vi "GEA3 HexStringToBoolean.vi"(2 "Hex String":string) -> (0 "Boolean":bool, 1 "decimal integer string":string)   [LabVIEW 2020]
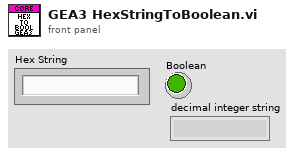
[diagram p1: front panel]
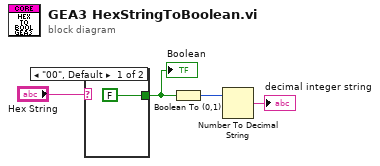
[diagram p0: block diagram]
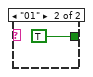
[diagram p2: hidden frame]
diagram:
  n1 = case shown="\"00\", Default" "Hex String" {
    tunnel: [FALSE ("Eco Wash") TRUE ("Eco Wash")] -> w3
    frame "00", Default {
    }
    frame "01" {
    }
  }
  "Boolean" <- w3
  n2 = Boolean To (0,1)(Boolean=w3) -> (0, 1=w2:i16)
  n3 = Number To Decimal String(number=w2) -> (decimal integer string=→"decimal integer string":string)  [unwired: 1 in]
